vi "HTTP tests.vi"() -> ()   [LabVIEW 2014]
uses:
  <vilib>/httpClient/LabVIEWHTTPClient.lvlib
panel:
  out "error out":errorcluster
  out "headers":string
  out "body":string
  in  "url":string="kirsch.dyndns.tv:8083/videostream.cgi?user=kirsch&pwd=QA2xEDcZvmuE"
  in  "password":string
  in  "username":string="kirsch"
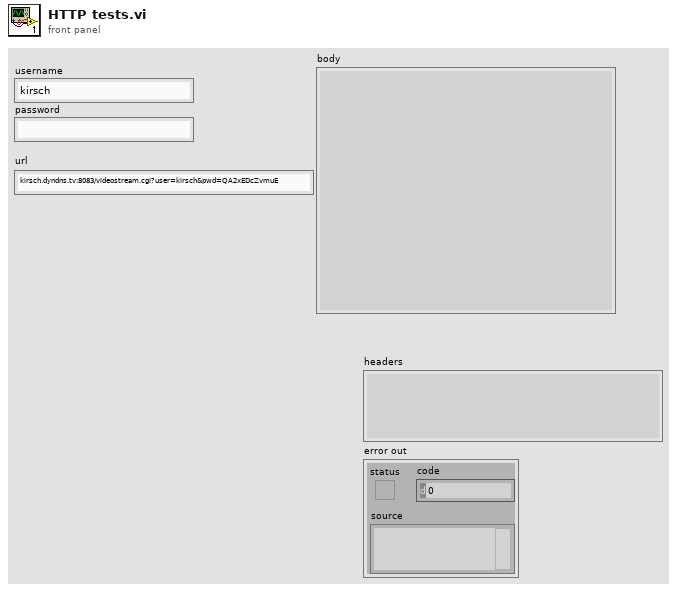
[diagram p1: front panel]
types:
  T1 = typedef "LabVIEWHTTPClient.lvlib/ClientHandle.ctl" = refnum<k1>
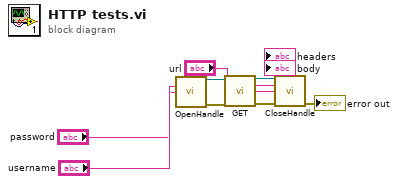
[diagram p0: block diagram]
diagram:
  n1 = call <vilib>:"OpenHandle.vi"("username"="username", "password"="password") -> ("client handle out"=w10:T1, "error out"=w9:errorcluster)  [unwired: 12 in]
  n2 = call <vilib>:"GET.vi"("client handle"=w10, "url"="url", "error in (no error)"=w9) -> ("client handle out"=w8:T1, "headers"=→"headers":string, "body"=→"body":string, "error out"=w7:errorcluster)  [unwired: 9 in]
  n3 = call <vilib>:"CloseHandle.vi"("client handle"=w8, "error in (no error)"=w7) -> ("error out"=→"error out":errorcluster)  [unwired: 13 in]
